vi "EF_GetFeaturesCSP.vi"(8 "error in (no error)":errorcluster, 10 "CSP filter file":path, 11 "Array Of Waveforms in":waveform(dbl)[](array[waveform])) -> (0 "error out":errorcluster, 3 "Array Of Waveforms out":waveform(dbl)[](array[waveform]))   [LabVIEW 2016, in "Feature Extraction.lvlib"]
uses:
  <vilib>/Analysis/Matrix/Datatypes/RealMatrix.ctl
  <vilib>/Analysis/baseanly.llb/Real A x B.vi
  <vilib>/Analysis/Matrix/Numeric/Conversions/Array To Matrix - RA2.vi
  <vilib>/Analysis/Matrix/Numeric/Conversions/Matrix To Array - RM.vi
  Feature Extraction.lvlib
  <vilib>/Analysis/Matrix/NI_Matrix.lvlib
  <vilib>/Analysis/NI_AALBase.lvlib
panel:
  # "This VI is a part of BCI Design library, http://www.ru-bci.org \nCopyright © 2020, Sotnikov Peter, All rights reserved. License: GNU GPLv3"
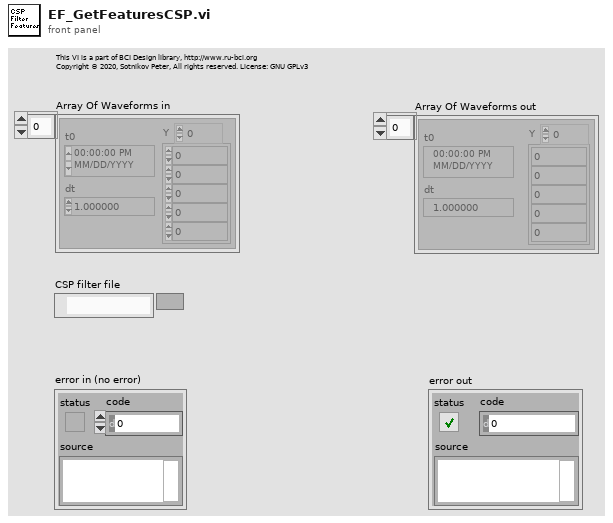
[diagram p1: front panel]
types:
  T1 = typedef "NI_Matrix.lvlib/RealMatrix.ctl" = dbl[][]
  T2 = enum16{"big-endian, network order", "native, host order", "little-endian"}
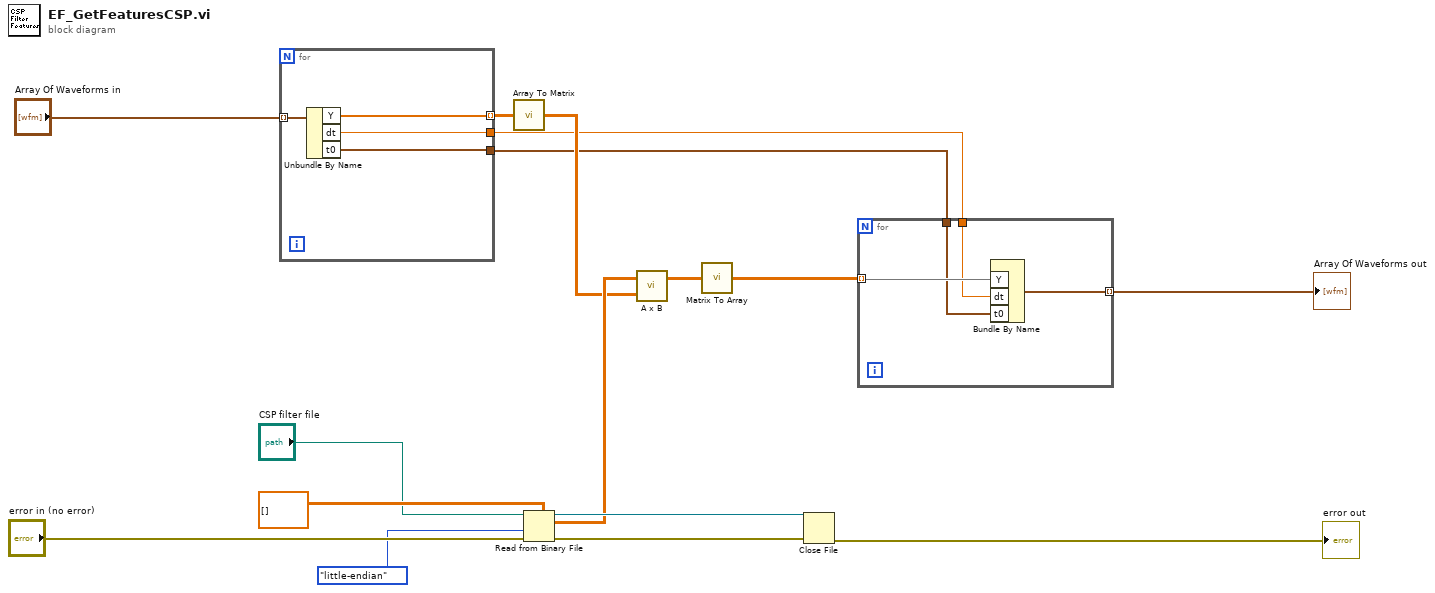
[diagram p0: block diagram]
diagram:
  n1 = for {
    tunnel: "Array Of Waveforms in" -> [w20] mode=indexing
    tunnel: [w19] -> w9 mode=indexing
    tunnel: [w18] -> w3
    tunnel: [w17] -> w2
    n2 = Unbundle By Name(w20) -> ("Y"=w19:dbl[], "dt"=w18:dbl, "t0"=w17:timestamp)
  }
  n3 = call-poly <vilib>:"Array To Matrix.vi"("Real 2D Array"=w9) -> ("Real Matrix"=w7:T1)
  n4 = Read from Binary File(5:T1 [] ("appended array"), 8:"error in (no error)", 9:T2."little-endian" ("byte order (0:big-endian, network order)"), 11:"CSP filter file") -> (0:w13:errorcluster, 2:w8:T1, 3:w11:refnum<file>)  [unwired: 2 in, 1 out]
  n5 = call-poly <vilib>:"A x B.vi"("B"=w7, "A"=w8) -> ("A x B"=w6:T1)  [unwired: 1 out]
  n6 = call-poly <vilib>:"Matrix To Array.vi"("Real Matrix"=w6) -> ("Real 2D Array"=w5:dbl[][])
  n7 = Close File(refnum=w11, error in=w13) -> (error out=→"error out":errorcluster)  [unwired: 1 out]
  n8 = for {
    tunnel: w5 -> [w24] mode=indexing
    tunnel: w3 -> [w23]
    tunnel: w2 -> [w22]
    tunnel: [w21] -> w1 mode=indexing
    n9 = Bundle By Name("Y"=w24, "dt"=w23, "t0"=w22) -> (w21:waveform(dbl))  [unwired: 1 in]
  }
  "Array Of Waveforms out" <- w1
